vi "Teleop.vi"(10 "Match Info":T1={"Autonomous Elapsed Seconds"=0.0, "TeleOp Elapsed Seconds"=0.0, "Disabled Elapsed Seconds"=0.0, "Visited Autonomous"=FALSE, "Visited TeleOp"=FALSE, "Visited Disabled"=FALSE, "Autonomous Settings"={"Autonomous Style"=enum."Independent", "VI Refnum"=refnum}}, 11 "Call Context":T2) -> ()   [LabVIEW 2013]
doc: "This VI is called for each TeleOp packet received from the DS where the robot is not disabled. It is often used to read from the joysticks and update I/O or to update setpoints for timed control loops. It should complete and return within 20 milliseconds or it may miss DS packets."
uses:
  <vilib>/Rock Robotics/WPI/DriverStation/WPI_DriverStationDerivedRobotMode.ctl
  <vilib>/Rock Robotics/WPI/DriverStation/WPI_DriverStationMatch Info.ctl
  <vilib>/Rock Robotics/WPI/Solenoid/WPI_SolenoidValue.ctl
  Specials/Global Data.vi
  <vilib>/Rock Robotics/WPI/Joystick/WPI_JoystickGetSetRefNum.vi
panel:
  in  "Xbox Controller?":bool
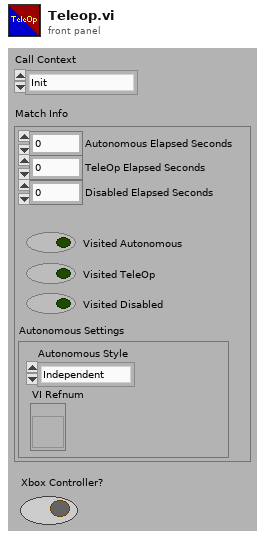
[diagram p1: front panel]
types:
  T1 = typedef "WPI_DriverStationMatch Info.ctl" = cluster{"Autonomous Elapsed Seconds":dbl, "TeleOp Elapsed Seconds":dbl, "Disabled Elapsed Seconds":dbl, "Visited Autonomous":bool, "Visited TeleOp":bool, "Visited Disabled":bool, "Autonomous Settings":cluster{"Autonomous Style":enum16{"Iterative", "Independent"}, "VI Refnum":refnum<vi>}}
  T2 = typedef "WPI_DriverStationDerivedRobotMode.ctl" = enum16{"Init", "Execute", "Stop"}
  T3 = typedef "WPI_JoystickDevRef.ctl" = cluster{"Device":T4}
  T4 = typedef "WPI_JoystickDeviceEnum.ctl" = enum16{"USB 1", "USB 2", "USB 3", "USB 4", "Kinect 1", "Kinect 2"}
  T5 = cluster{"axis 1 (x)":dbl, "axis 2 (y)":dbl, "axis 3 (throttle)":dbl, "axis 4":dbl, "axis 5":dbl, "axis 6":dbl}
  T6 = typedef "WPI_SolenoidValue.ctl" = enum16{"Off", "On", "Forward", "Reverse"}
  T7 = typedef "WPI_JoystickButtonState.ctl" = cluster{"Button 1":bool, "Button 2":bool, "Button 3":bool, "Button 4":bool, "Button 5":bool, "Button 6":bool, "Button 7":bool, "Button 8":bool, "Button 9":bool, "Button 10":bool, "Button 11":bool, "Button 12":bool}
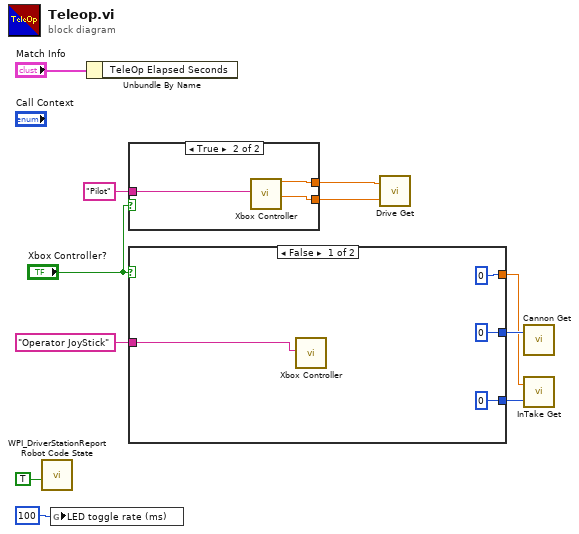
[diagram p0: block diagram]
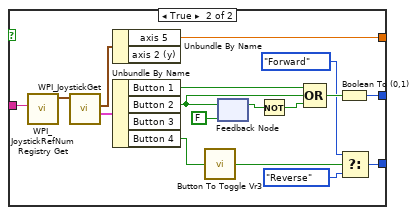
[diagram p2: hidden frame]
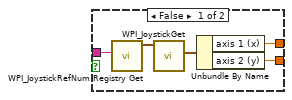
[diagram p3: hidden frame]
diagram:
  n1 = call <vilib>:"WPI_DriverStationReport Robot Code State.vi"("TeleOp"=TRUE ("Autonomous")) -> ()  [unwired: 10 in, 1 out]
  n2 = global write "Global Data.vi" "LED toggle rate (ms)"(u32 100 ("LED ms toggle rate")) -> ()
  n3 = Unbundle By Name("Match Info") -> ()  [unwired: 1 out]
  n4 = case shown="True" "Xbox Controller?" {
    tunnel: "Pilot" ("refnum name") -> [w15 w19]
    tunnel: [w13 w18] -> w7
    tunnel: [w12 w17] -> w6
    frame False {
      n5 = call <vilib>:"WPI_JoystickRefNum Registry Get.vi"("refnum name"=w15) -> ("JoystickDevRef"=w16:T3)  [unwired: 9 in, 1 out]
      n6 = call <vilib>:"WPI_JoystickGet.vi"("JoystickDevRef"=w16) -> ("Axes"=w14:T5)  [unwired: 4 in, 2 out]
      n7 = Unbundle By Name(w14) -> ("axis 1 (x)"=w13:dbl, "axis 2 (y)"=w12:dbl)
    }
    frame True {
      n8 = call "Xbox Controller.vi"("Joystick Name"=w19) -> ("Left Stick Y"=w18:dbl, "Right Stick Y"=w17:dbl)  [unwired: 3 in, 14 out]
    }
  }
  n9 = case shown="False" "Xbox Controller?" {
    tunnel: "Operator JoyStick" ("refnum name") -> [w20 w37]
    tunnel: [0 w36] -> w2
    tunnel: [0 w26] -> w3
    tunnel: [0 w33] -> w4
    frame False {
      n10 = call "Xbox Controller.vi"("Joystick Name"=w20) -> ()  [unwired: 3 in, 16 out]
    }
    frame True {
      n11 = call <vilib>:"WPI_JoystickRefNum Registry Get.vi"("refnum name"=w37) -> ("JoystickDevRef"=w38:T3)  [unwired: 9 in, 1 out]
      n12 = call <vilib>:"WPI_JoystickGet.vi"("JoystickDevRef"=w38) -> ("Buttons"=w39:T7, "Axes"=w40:T5)  [unwired: 4 in, 1 out]
      n13 = Unbundle By Name(w40) -> ("axis 5"=w36:dbl)  [unwired: 1 out]
      n14 = Unbundle By Name(w39) -> ("Button 1"=w32:bool, "Button 2"=w31:bool, "Button 4"=w28:bool)  [unwired: 1 out]
      n15 = call "Button To Toggle Vr3.vi"("InValue"=w28) -> ("Result"=w27:bool)
      n16 = feedback-in #1(w31) -> ()
      n17 = feedback #1(FALSE ("Button 2")) -> (w35:bool)
      n18 = Not(x=w35) -> (.not. x?=w30:bool)
      n19 = Compound Arithmetic op=OR(w32, w31, w30) -> (w29:bool)
      n20 = Boolean To (0,1)(Boolean=w29) -> (0, 1=w33:i16)
      n21 = Select(t=WPI_SolenoidValue."Forward" ("MoveArm"), s=w27, f=WPI_SolenoidValue."Reverse" ("MoveArm")) -> (s? t:f=w26:T6)
    }
  }
  n22 = call "Drive Get.vi"("Y"=w6, "X"=w7) -> ()  [unwired: 1 in]
  n23 = call "Cannon Get.vi"("Solenoid"=w4) -> ()  [unwired: 2 in]
  n24 = call "InTake Get.vi"("MoveArm"=w3, "TakeBall"=w2) -> ()  [unwired: 1 in]
